vi "RichToFlatnixnet_grpc_ReadFrameRequest.vi"(5 "OutputClusterType":T1, 11 "InputCluster":T5) -> (3 "OutputCluster":T1)   [LabVIEW 2024, in "grpc-xnet_client.lvlib"]
uses:
  grpc-xnet_client.lvlib
  nixnet_grpc_ReadFrameRequest_protocol_enum/nixnet_grpc_ReadFrameRequest_protocol_enum.lvclass
  nixnet_grpc_ReadFrameRequest_timeout_enum/nixnet_grpc_ReadFrameRequest_timeout_enum.lvclass
  nixnet_grpc_ReadFrameRequest_protocol_enum/nixnet_grpc_ReadFrameRequest_protocol_enum.lvclass/nixnet_grpc_ReadFrameRequest_protocol_enum.ctl
  nixnet_grpc_ReadFrameRequest_timeout_enum/nixnet_grpc_ReadFrameRequest_timeout_enum.lvclass/nixnet_grpc_ReadFrameRequest_timeout_enum.ctl
  nixnet_grpc_TimeOut.ctl
  nixnet_grpc_Protocol.ctl
  nidevice_grpc_Session_Flat.ctl
  nixnet_grpc_ReadFrameRequest_Flat.ctl
  nidevice_grpc_Session.ctl
  nixnet_grpc_ReadFrameRequest.ctl
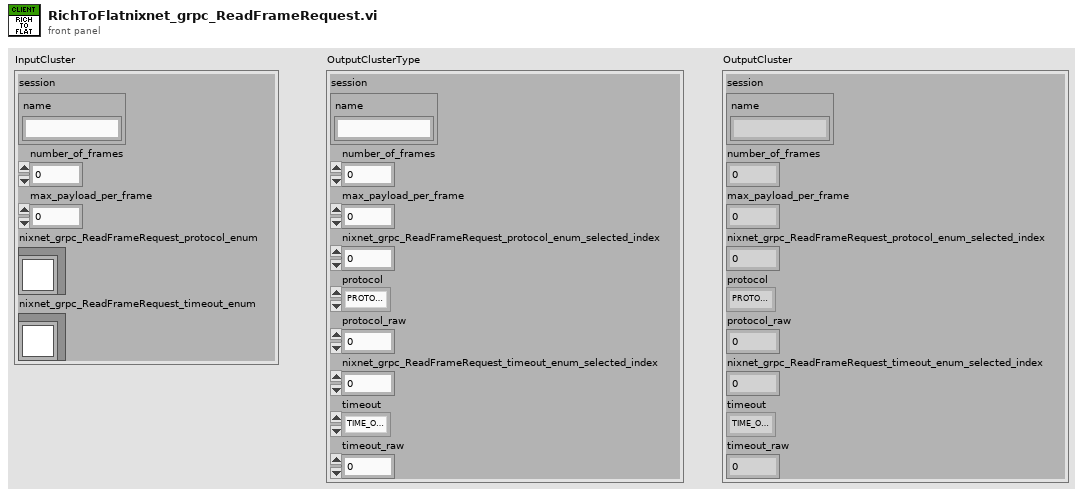
[diagram p1: front panel]
types:
  T1 = typedef "grpc-xnet_client.lvlib/nixnet_grpc_ReadFrameRequest_Flat.ctl" = cluster{"session":T2, "number_of_frames":i32, "max_payload_per_frame":u32, "nixnet_grpc_ReadFrameRequest_protocol_enum_selected_index":i32, "protocol":T3, "protocol_raw":u32, "nixnet_grpc_ReadFrameRequest_timeout_enum_selected_index":i32, "timeout":T4, "timeout_raw":dbl}
  T2 = typedef "grpc-xnet_client.lvlib/nidevice_grpc_Session_Flat.ctl" = cluster{"name":string}
  T3 = typedef "grpc-xnet_client.lvlib/nixnet_grpc_Protocol.ctl" = enum32{"PROTOCOL_UNSPECIFIED", "PROTOCOL_CAN", "PROTOCOL_LIN", "PROTOCOL_FLEX_RAY", "PROTOCOL_J1939", "PROTOCOL_ENET"}
  T4 = typedef "grpc-xnet_client.lvlib/nixnet_grpc_TimeOut.ctl" = enum32{"TIME_OUT_NONE", "TIME_OUT_INFINITE"}
  T5 = typedef "grpc-xnet_client.lvlib/nixnet_grpc_ReadFrameRequest.ctl" = cluster{"session":T6, "number_of_frames":i32, "max_payload_per_frame":u32, "nixnet_grpc_ReadFrameRequest_protocol_enum":refnum<class "nixnet_grpc_ReadFrameRequest_protocol_enum.lvclass">, "nixnet_grpc_ReadFrameRequest_timeout_enum":refnum<class "nixnet_grpc_ReadFrameRequest_timeout_enum.lvclass">}
  T6 = typedef "grpc-xnet_client.lvlib/nidevice_grpc_Session.ctl" = cluster{"name":string}
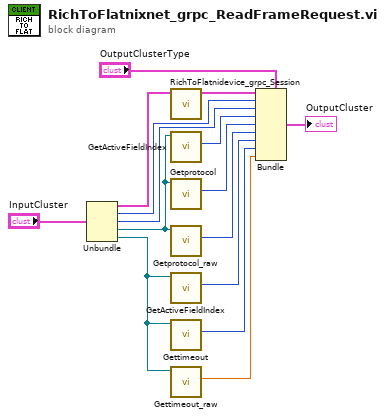
[diagram p0: block diagram]
diagram:
  n1 = Unbundle "Unbundle"("InputCluster") -> ("session"=w12:T6, "number_of_frames"=w10:i32, "max_payload_per_frame"=w9:u32, "nixnet_grpc_ReadFrameRequest_protocol_enum"=w8:refnum<class "nixnet_grpc_ReadFrameRequest_protocol_enum.lvclass">, "nixnet_grpc_ReadFrameRequest_timeout_enum"=w4:refnum<class "nixnet_grpc_ReadFrameRequest_timeout_enum.lvclass">)
  n2 = call "RichToFlatnidevice_grpc_Session.vi"("InputCluster"=w12) -> ("OutputCluster"=w11:T2)  [unwired: 10 in]
  n3 = call "GetActiveFieldIndex.vi"("OneOfTemplate in"=w8) -> ("Active Field Index"=w7:i32)  [unwired: 8 in, 2 out]
  n4 = call "Getprotocol.vi"("OneOfTemplate in"=w8) -> ("Get_Val"=w6:T3)  [unwired: 8 in, 2 out]
  n5 = call "Getprotocol_raw.vi"("OneOfTemplate in"=w8) -> ("Get_Val"=w5:u32)  [unwired: 8 in, 2 out]
  n6 = call "GetActiveFieldIndex.vi"("OneOfTemplate in"=w4) -> ("Active Field Index"=w3:i32)  [unwired: 8 in, 2 out]
  n7 = call "Gettimeout.vi"("OneOfTemplate in"=w4) -> ("Get_Val"=w2:T4)  [unwired: 8 in, 2 out]
  n8 = call "Gettimeout_raw.vi"("OneOfTemplate in"=w4) -> ("Get_Val"=w1:dbl)  [unwired: 8 in, 2 out]
  n9 = Bundle "Bundle"(cluster="OutputClusterType", "session"=w11, "number_of_frames"=w10, "max_payload_per_frame"=w9, "nixnet_grpc_ReadFrameRequest_protocol_enum_selected_index"=w7, "protocol"=w6, "protocol_raw"=w5, "nixnet_grpc_ReadFrameRequest_timeout_enum_selected_index"=w3, "timeout"=w2, "timeout_raw"=w1) -> (→"OutputCluster":T1)
